vi "DeSync.vi"(8 "error in":errorcluster, 10 "inputData":cdb[](array[numeric]), 11 "Path In":path) -> (0 "error out":errorcluster, 1 "modScCorr":dbl[](array[numeric]) format="%#_13g", 2 "out_data":cdb[](array[numeric]), 3 "Path Out":path)   [LabVIEW 2015]
panel:
  out "数值":i32
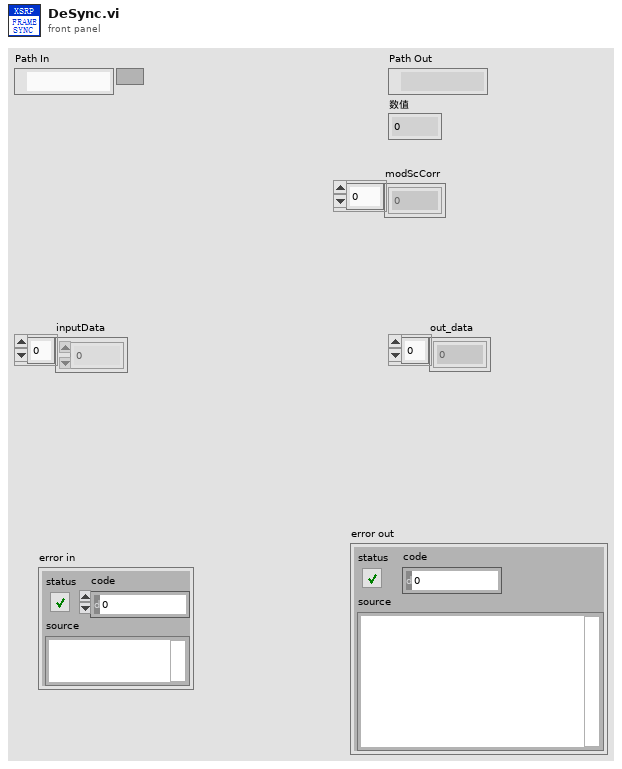
[diagram p1: front panel]
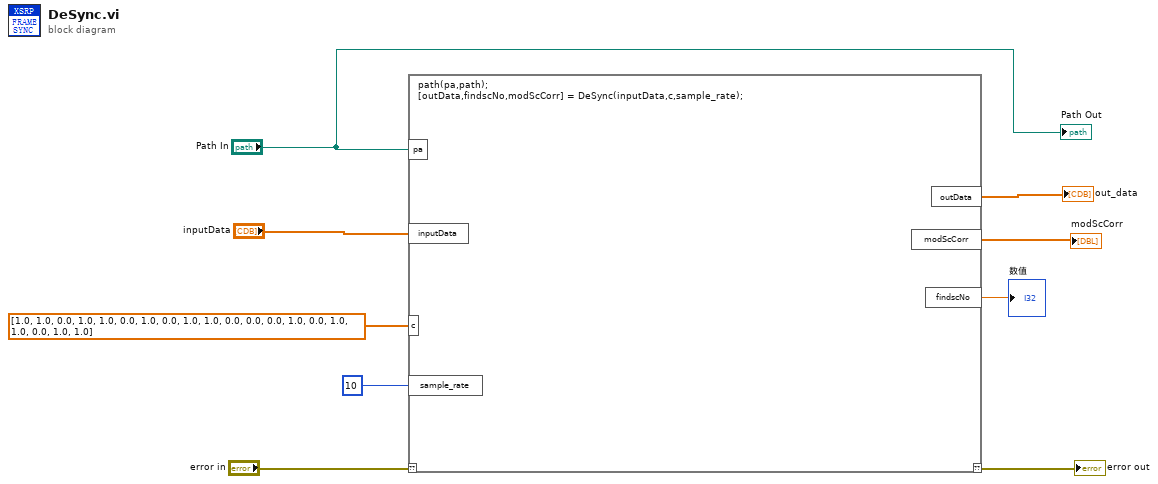
[diagram p0: block diagram]
diagram:
  n1 = script code="path(pa,path);\n[outData,findscNo,modScCorr] = DeSync(inputData,c,sample_rate);"("??"="error in", "pa"="Path In", "inputData"="inputData", "c"=dbl[] [1.0, 1.0, 0.0, 1.0, 1.0, 0.0, 1.0, 0.0, 1.0, 1.0, 0.0, 0.0, 0.0, 1.0, 0.0, 1.0, 1.0, 0.0, 1.0, 1.0], "sample_rate"=10) -> ("??"=→"error out":errorcluster, "outData"=→"out_data":cdb[], "findscNo"=→"数值":dbl, "modScCorr"=→"modScCorr":dbl[])
  "Path Out" <- "Path In"
